vi "Obtain_User_Event.vi"(8 "error in (no error)":errorcluster, 11 "Name":string) -> (0 "error out":errorcluster, 3 "user event out":refnum<user-event>)   [LabVIEW 2014, in "User_Event_Library.lvlib"]
uses:
  User_Event_Library.lvlib
  TypeDef.ctl
panel:
  # "將Name接腳設定為必接"
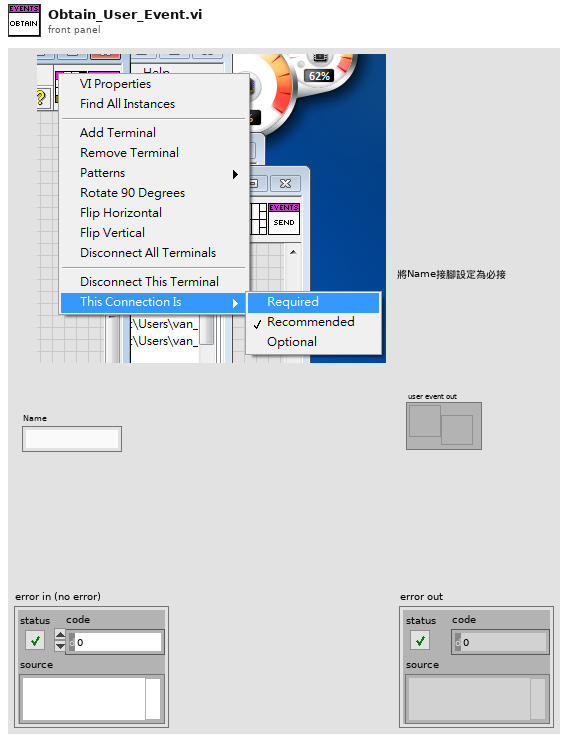
[diagram p1: front panel]
types:
  T1 = typedef "User_Event_Library.lvlib/TypeDef.ctl" = cluster{"Command":string, "Data":variant}
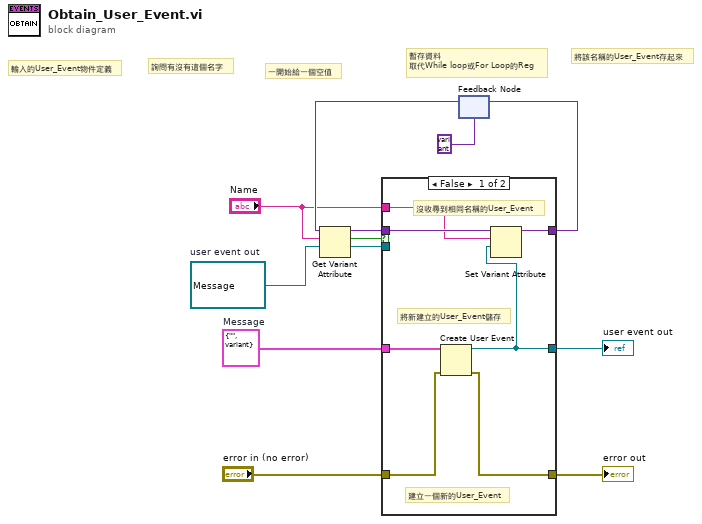
[diagram p0: block diagram]
diagram:
  w1 = refnum<user-event> refnum  # user event out
  w10 = T1 {"Command"="", "Data"=variant}  # Message
  # "將該名稱的User_Event存起來"
  # "輸入的User_Event物件定義"
  # "詢問有沒有這個名字"
  # "一開始給一個空值"
  # "暫存資料\n取代While loop或For Loop的Reg"
  n1 = feedback #1(variant) -> (w7:variant)
  n2 = Get Variant Attribute(Variant=w7, name="Name", default value (empty Variant)=w1) -> (duplicate Variant=w5:variant, found=w6:bool, value=w2:refnum<user-event>)  [unwired: 1 in, 1 out]
  n3 = case shown="False" w6 {
    tunnel: "error in (no error)" -> [w19 w21]
    tunnel: [w18 w21] -> w11
    tunnel: w10 -> [w17 _]
    tunnel: [w13 w20] -> w9
    tunnel: w5 -> [w16 w22]
    tunnel: "Name" -> [w15 _]
    tunnel: [w14 w22] -> w3
    tunnel: w2 -> [_ w20]
    frame False {
      # "將新建立的User_Event儲存"
      # "建立一個新的User_Event"
      # "沒收尋到相同名稱的User_Event"
      n4 = Create User Event(user event datatype=w17, error in=w19) -> (user event=w13:refnum<user-event>, error out=w18:errorcluster)
      n5 = Set Variant Attribute(Variant=w16, name=w15, value=w13) -> (Variant out=w14:variant)  [unwired: 1 in, 2 out]
    }
    frame True {
      # "有搜尋到相同名稱的\nUser_Events"
    }
  }
  "error out" <- w11
  "user event out" <- w9
  n6 = feedback-in #1(w3) -> ()
